vi "RobotGlobal.vi"() -> ()   [LabVIEW 2019]
uses:
  TypeDefs/RobotObjects.ctl
  Classes/Pnematics control/Pneumatics.lvclass
  Classes/Vision/Vision.lvclass
  Classes/Joysticks/Joysticks.lvclass
  Classes/Elevator/Elevator.lvclass
  Classes/Hatch/Hatch.lvclass
  Classes/Cargo/Cargo.lvclass
  Classes/Drive/Tank Drive/Tank Drive.lvclass
  Classes/DriveOld/Drive.lvclass
  Classes/Robot/Robot.lvclass
  Classes/Control Panel/Control Panel.lvclass
  Classes/Climber/Climber.lvclass
  Classes/Turret/Turret.lvclass
  Classes/PowerCellHandler/Power Cell Handler.lvclass
  TypeDefs/Falcon Temperatures.ctl
panel:
  in  "Falcon Temperatures":T1
  in  "CodeConfigFile":path
  in  "RobotData":T2
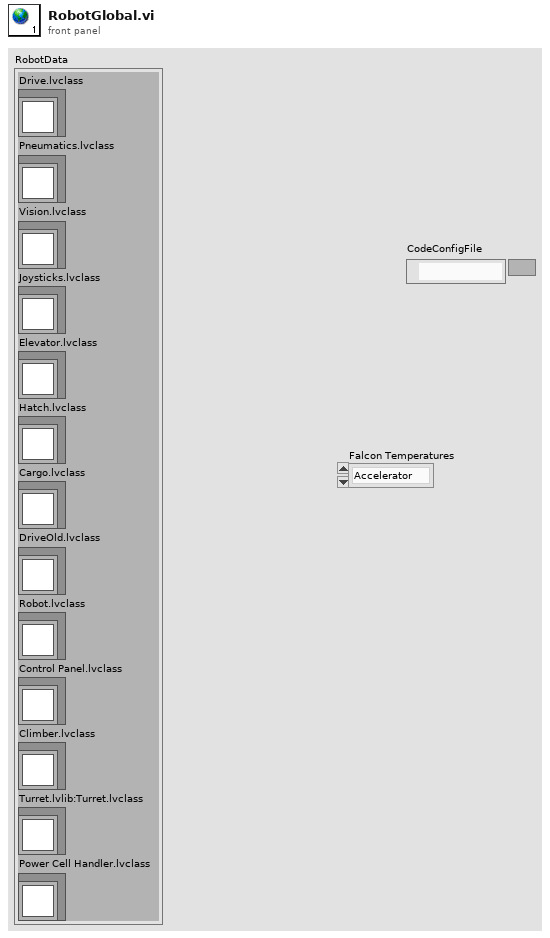
[diagram p1: front panel]
types:
  T1 = typedef "Falcon Temperatures.ctl" = enum16{"Accelerator", "Flywheel", "Right follow", "Right lead", "Left follow", "Left lead"}
  T2 = typedef "RobotObjects.ctl" = cluster{"Drive.lvclass":refnum<class "Tank Drive.lvclass">, "Pneumatics.lvclass":refnum<class "Pneumatics.lvclass">, "Vision.lvclass":refnum<class "Vision.lvclass">, "Joysticks.lvclass":refnum<class "Joysticks.lvclass">, "Elevator.lvclass":refnum<class "Elevator.lvclass">, "Hatch.lvclass":refnum<class "Hatch.lvclass">, "Cargo.lvclass":refnum<class "Cargo.lvclass">, "DriveOld.lvclass":refnum<class "Drive.lvclass">, "Robot.lvclass":refnum<class "Robot.lvclass">, "Control Panel.lvclass":refnum<class "Control Panel.lvclass">, "Climber.lvclass":refnum<class "Climber.lvclass">, "Turret.lvlib:Turret.lvclass":refnum<class "Turret.lvclass">, "Power Cell Handler.lvclass":refnum<class "Power Cell Handler.lvclass">}
diagram:
